vi "Write (De-)Embed.vi"(10 "(De-)Embed":T1(array[cluster])=[{"enabled"=FALSE, "De-embed"=TRUE, "Swap Ports Left"=FALSE, "De-embedding file"=path ""}, {"enabled"=FALSE, "De-embed"=TRUE, "Swap Ports Left"=FALSE, "De-embedding file"=path ""}], 11 "S Parameter in":refnum<class "S Parameter.lvclass">) -> (3 "S Parameter out":refnum<class "S Parameter.lvclass">)   [LabVIEW 2020, in "S Parameter.lvclass"]
uses:
  S Parameter.lvclass
  S Parameter.lvclass/S Parameter.ctl
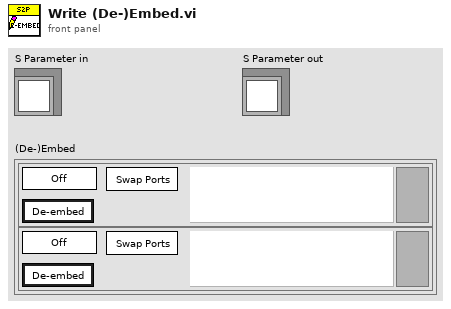
[diagram p1: front panel]
types:
  T1 = cluster{"enabled":bool, "De-embed":bool, "Swap Ports Left":bool, "De-embedding file":path}[]
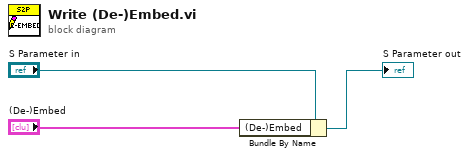
[diagram p0: block diagram]
diagram:
  n1 = Bundle By Name(cluster="S Parameter in", "(De-)Embed"="(De-)Embed") -> (→"S Parameter out":refnum<class "S Parameter.lvclass">)
